vi "sub_GSlam_cal-edge.vi"(11 "in":T3) -> (3 "edge out":T1={"e"=[[0.04000000000000001]], "omega"=[[0.04000000000000001]], "d1"=0.0, "d2"=0.0, "yaw1"=0.0, "yaw2"=0.0, "angle1"=0.0, "angle2"=0.0, "id1"=0, "id2"=0})   [LabVIEW 2019]
uses:
  Ctrl/slam_edge.ctl
  <vilib>/Analysis/Matrix/Datatypes/RealMatrix.ctl
  <vilib>/Analysis/coordinate.llb/Euler Rotation Order.ctl
  <vilib>/Analysis/Matrix/Numeric/Conversions/Array To Matrix - RA.vi
  <vilib>/Analysis/Matrix/Numeric/Conversions/Array To Matrix - RA2.vi
  <vilib>/Analysis/Matrix/Numeric/Multiply/Multiply - RM,RM.vi
  <vilib>/Analysis/Matrix/Numeric/Add/Add - RM,RM.vi
  <vilib>/Analysis/baseanly.llb/Real Inverse Matrix.vi
  <vilib>/Analysis/Matrix/NI_Matrix.lvlib
  <vilib>/Analysis/NI_AALPro.lvlib
  <vilib>/Analysis/NI_AALBase.lvlib
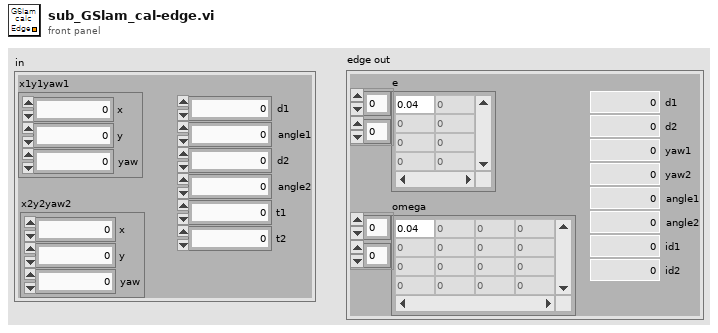
[diagram p1: front panel]
types:
  T1 = typedef "slam_edge.ctl" = cluster{"e":T2, "omega":T2, "d1":dbl, "d2":dbl, "yaw1":dbl, "yaw2":dbl, "angle1":dbl, "angle2":dbl, "id1":i32, "id2":i32}
  T2 = typedef "NI_Matrix.lvlib/RealMatrix.ctl" = dbl[][]
  T3 = cluster{"x1y1yaw1":cluster{"x":dbl, "y":dbl, "yaw":dbl}, "x2y2yaw2":cluster{"x":dbl, "y":dbl, "yaw":dbl}, "d1":dbl, "angle1":dbl, "d2":dbl, "angle2":dbl, "t1":i32, "t2":i32}
  T4 = typedef "NI_AALPro.lvlib/Euler Rotation Order.ctl" = u16
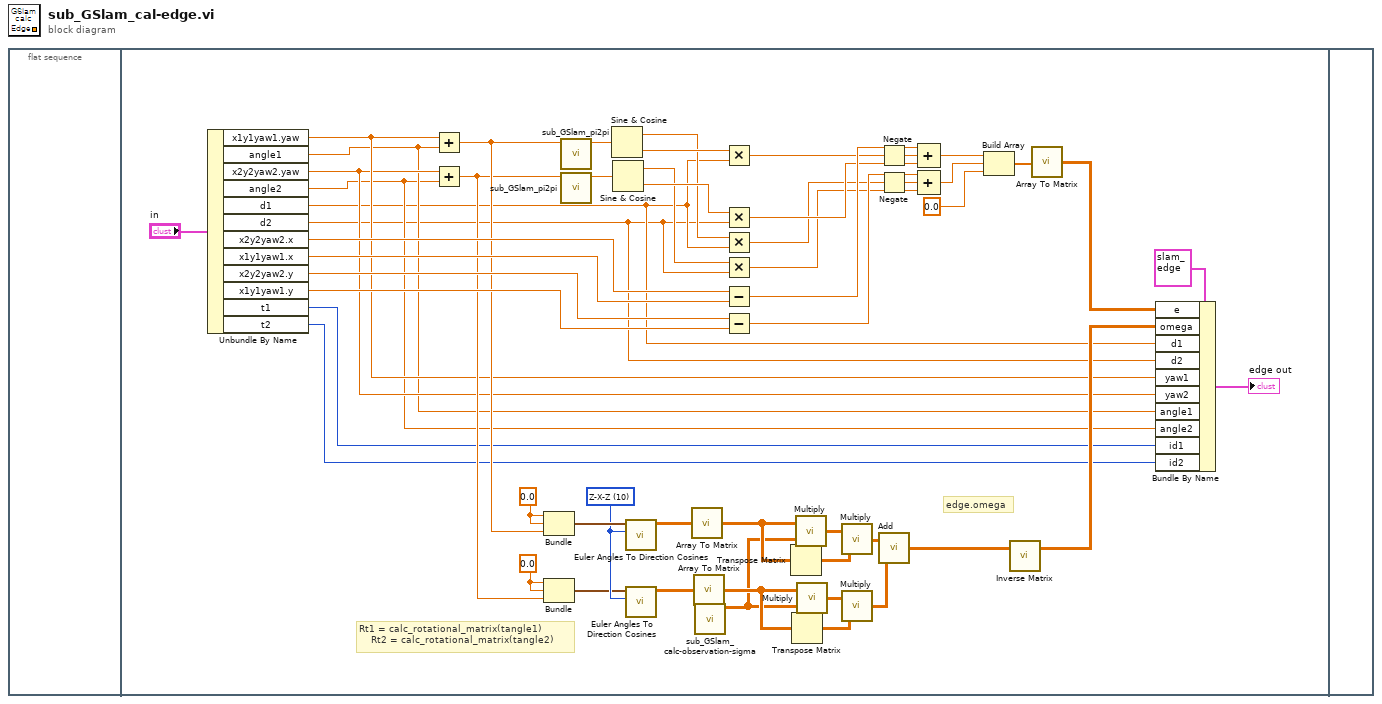
[diagram p0: block diagram]
diagram:
  n1 = flat-sequence {
    frame #0 {
    }
    frame #1 {
      w25 = T4 10 items=["X-Y-Z", "X-Z-Y", "Y-X-Z", "Y-Z-X", "Z-X-Y", "Z-Y-X", "X-Y-X", "X-Z-X", "Y-X-Y", "Y-Z-Y", "Z-X-Z", "Z-Y-Z"] ("rotation order")
      w28 = 0.0 ("원소")
      w30 = 0.0 ("원소")
      # "edge.omega"
      # "Rt1 = calc_rotational_matrix(tangle1)\n    Rt2 = calc_rotational_matrix(tangle2)"
      n2 = Unbundle By Name("in") -> ("x1y1yaw1.yaw"=w10:dbl, "angle1"=w8:dbl, "x2y2yaw2.yaw"=w9:dbl, "angle2"=w7:dbl, "d1"=w6:dbl, "d2"=w5:dbl, "x2y2yaw2.x"=w47:dbl, "x1y1yaw1.x"=w46:dbl, "x2y2yaw2.y"=w42:dbl, "x1y1yaw1.y"=w41:dbl, "t1"=w4:i32, "t2"=w3:i32)
      n3 = Add(x=w10, y=w8) -> (x+y=w29:dbl)
      n4 = Add(x=w9, y=w7) -> (x+y=w27:dbl)
      n5 = Bundle("원소"=w30, "원소"=w30, w29) -> (w26:cluster{"원소":dbl, "원소":dbl, dbl})  [unwired: 1 in]
      n6 = Bundle("원소"=w28, "원소"=w28, w27) -> (w24:cluster{"원소":dbl, "원소":dbl, dbl})  [unwired: 1 in]
      n7 = call "sub_GSlam_pi2pi.vi"("angle"=w29) -> ("result"=w53:dbl)  [unwired: 10 in]
      n8 = call "sub_GSlam_pi2pi.vi"("angle"=w27) -> ("result"=w52:dbl)  [unwired: 10 in]
      n9 = Sine & Cosine(0:w53) -> (1:w49:dbl, 2:w51:dbl)
      n10 = Sine & Cosine(0:w52) -> (1:w48:dbl, 2:w50:dbl)
      n11 = call <vilib>:"Euler Angles To Direction Cosines.vi"("rotation order"=w25, "Euler Angles"=w26) -> ("Direction Cosines"=w23:dbl[][])  [unwired: 8 in, 1 out]
      n12 = call <vilib>:"Euler Angles To Direction Cosines.vi"("rotation order"=w25, "Euler Angles"=w24) -> ("Direction Cosines"=w17:dbl[][])  [unwired: 8 in, 1 out]
      n13 = call-poly <vilib>:"Array To Matrix.vi"("Real 2D Array"=w23) -> ("Real Matrix"=w20:T2)
      n14 = call-poly <vilib>:"Array To Matrix.vi"("Real 2D Array"=w17) -> ("Real Matrix"=w16:T2)
      n15 = call "sub_GSlam_calc-observation-sigma.vi"() -> ("sigma"=w15:T2)  [unwired: 11 in]
      n16 = Multiply ("tmp1")(x=w51, y=w6) -> (x*y=w44:dbl)
      n17 = Multiply ("tmp2")(x=w50, y=w5) -> (x*y=w40:dbl)
      n18 = Multiply ("tmp3")(x=w49, y=w6) -> (x*y=w37:dbl)
      n19 = Multiply ("tmp4")(x=w48, y=w5) -> (x*y=w36:dbl)
      n20 = Subtract(x=w47, y=w46) -> (x-y=w45:dbl)
      n21 = Subtract(x=w42, y=w41) -> (x-y=w38:dbl)
      n22 = Transpose Matrix(1:w20) -> (0:w21:T2)
      n23 = Transpose Matrix(1:w16) -> (0:w19:T2)
      n24 = call-poly <vilib>:"Multiply.vi"("Real Matrix B"=w15, "Real Matrix A"=w20) -> ("A * B"=w22:T2)
      n25 = call-poly <vilib>:"Multiply.vi"("Real Matrix B"=w15, "Real Matrix A"=w16) -> ("A * B"=w18:T2)
      n26 = call-poly <vilib>:"Multiply.vi"("Real Matrix B"=w21, "Real Matrix A"=w22) -> ("A * B"=w14:T2)
      n27 = call-poly <vilib>:"Multiply.vi"("Real Matrix B"=w19, "Real Matrix A"=w18) -> ("A * B"=w13:T2)
      n28 = Negate(x=w44) -> (-x=w43:dbl)
      n29 = Negate(x=w37) -> (-x=w39:dbl)
      n30 = call-poly <vilib>:"Add.vi"("Real Matrix B"=w13, "Real Matrix A"=w14) -> ("A + B"=w12:T2)
      n31 = Compound Arithmetic op=ADD(w45, w43, w40) -> (w35:dbl)
      n32 = Compound Arithmetic op=ADD(w38, w39, w36) -> (w34:dbl)
      n33 = Build Array(w35, w34, 0.0 ("원소")) -> (w32:dbl[])
      n34 = call-poly <vilib>:"Inverse Matrix.vi"("Input Matrix"=w12) -> ("Inverse Matrix"=w11:T2)  [unwired: 1 in, 1 out]
      n35 = call-poly <vilib>:"Array To Matrix.vi"("Real 1D Array"=w32) -> ("Real Matrix (Column Vector)"=w31:T2)
      n36 = Bundle By Name(cluster=T1 {"e"=[[0.0], [0.0], [0.0]], "omega"=[[0.0, 0.0, 0.0], [0.0, 0.0, 0.0], [-0.0, -0.0, 0.0]], "d1"=0.0, "d2"=0.0, "yaw1"=0.0, "yaw2"=0.0, "angle1"=0.0, "angle2"=0.0, "id1"=0, "id2"=0} ("pf-val out"), "e"=w31, "omega"=w11, "d1"=w6, "d2"=w5, "yaw1"=w10, "yaw2"=w9, "angle1"=w8, "angle2"=w7, "id1"=w4, "id2"=w3) -> (→"edge out":T1)
    }
    frame #2 {
    }
  }
